vi "CalcLines.vi"() -> ()   [LabVIEW 2012]
doc: "This VI takes in a set of angle value pairs as arrays and interpolates lines between them. It outputs arrays of slopes matched with intercepts matched with the indicies of a collection of angles which are used as follows:\n\nTo find a desired angle, iterate through the Angle/Indicies array until the current angle is greater than your desired angle. Then decrement your iterator by one to find the index of your desired slope and intercept.\n\n It works for any angle value pair with an angle input of 0 to 360 degrees. But if you're a stylistic purist don't give it a 0 or 360 degree input: it will still work, but it will have a weird double entry if you look at the output values."
uses:
  <vilib>/Analysis/NI_AALPro.lvlib
panel:
  out "Angles/Indicies":dbl[](array[numeric])
  out "Intercept":dbl[](array[numeric])
  out "Slope":dbl[](array[numeric])
  in  "Angles":dbl[](array[numeric])
  in  "Values":dbl[](array[numeric])
  # "Inputs"
  # "Outputs"
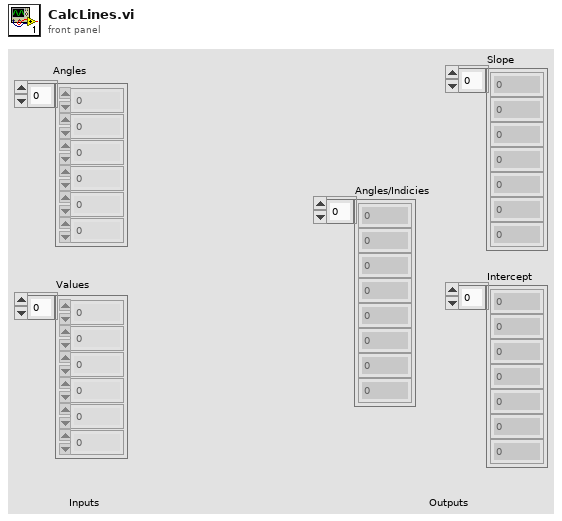
[diagram p1: front panel]
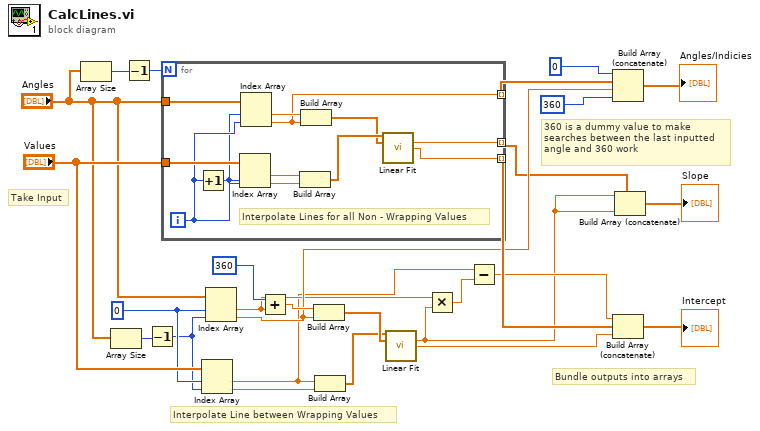
[diagram p0: block diagram]
diagram:
  w24 = 0
  # "Bundle outputs into arrays"
  # "360 is a dummy value to make\nsearches between the last inputted \nangle and 360 work"
  # "Interpolate Line between Wrapping Values"
  # "Take Input"
  n1 = Array Size(array="Angles") -> (size(s)=w27:i32)
  n2 = Array Size(array="Angles") -> (size(s)=w10:i32)
  n3 = Decrement(x=w27) -> (x-1=w26:i32)
  n4 = Decrement(x=w10) -> (x-1=w9:i32)
  n5 = for {
    N: w26 -> [_]
    tunnel: "Values" -> [w38]
    tunnel: "Angles" -> [w39]
    tunnel: [w31] -> w1 mode=indexing
    tunnel: [w30] -> w14 mode=indexing
    tunnel: [w28] -> w18 mode=indexing
    i -> [w37]
    # "Interpolate Lines for all Non - Wrapping Values"
    n6 = Increment(x=w37) -> (x+1=w36:i32)
    n7 = Index Array(array=w38, index #1=w36, index #2=w37) -> (element #1=w35:dbl, element #2=w34:dbl)
    n8 = Index Array(array=w39, index #1=w36, index #2=w37) -> (element #1=w29:dbl, element #2=w28:dbl)
    n9 = Build Array(w35, w34) -> (w33:dbl[])
    n10 = Build Array(w29, w28) -> (w32:dbl[])
    n11 = call <vilib>:"Linear Fit.vi"("Y"=w33, "X"=w32) -> ("slope"=w31:dbl, "intercept"=w30:dbl)  [unwired: 9 in, 3 out]
  }
  n12 = Index Array(array="Values", index #1=w24, index #2=w9) -> (element #1=w4:dbl, element #2=w22:dbl)
  n13 = Index Array(array="Angles", index #1=w24, index #2=w9) -> (element #1=w7:dbl, element #2=w12:dbl)
  n14 = Add(x=360, y=w7) -> (x+y=w23:dbl)
  n15 = Build Array(w23, w12) -> (w21:dbl[])
  n16 = Build Array(w4, w22) -> (w20:dbl[])
  n17 = call <vilib>:"Linear Fit.vi"("Y"=w20, "X"=w21) -> ("slope"=w3:dbl, "intercept"=w8:dbl)  [unwired: 9 in, 3 out]
  n18 = Multiply(x=w7, y=w3) -> (x*y=w6:dbl)
  n19 = Subtract(x=w4, y=w6) -> (x-y=w5:dbl)
  n20 = Build Array (concatenate)(0, w18, w12, 360) -> (→"Angles/Indicies":dbl[])
  n21 = Build Array (concatenate)(w5, w14, w8) -> (→"Intercept":dbl[])
  n22 = Build Array (concatenate)(w3, w1, w3) -> (→"Slope":dbl[])
